vi "Stop Core.vi"(10 "final error code":i32, 11 "DigitiserActor in":refnum<class "DigitiserActor.lvclass">) -> (3 "DigitiserActor out":refnum<class "DigitiserActor.lvclass">)   [LabVIEW 2019, in "DigitiserActor.lvlib" / "DigitiserActor.lvclass"]
doc: "(<B>Filename</B>: Actor Framework.lvlib:Actor.lvclass:Stop Core.vi)\n\nDefines what the actor does before it stops. Use the <B>final error code</B> input to determine whether the actor shut down in response to an error.\n\nBy default, this method passes the Stop message along to all auto-stop nested actors. A descendant class may override this method to define additional behavior, such as shutting down any processes the actor initiated in its override of the Actor Core method."
uses:
  DigitiserActor.lvclass
  <vilib>/ActorFramework/Actor/Actor.lvclass
  <vilib>/ActorFramework/Stop Msg/Stop Msg.lvclass
  C:/Program Files (x86)/National Instruments/LabVIEW 2019/vi.lib/ActorFramework/Actor/Actor.lvclass
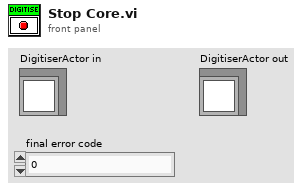
[diagram p1: front panel]
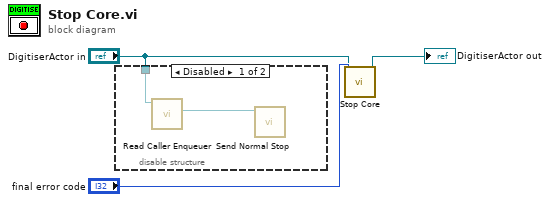
[diagram p0: block diagram]
diagram:
  n1 = disable-structure shown="Disabled" {
    disable-tunnel: "DigitiserActor in" -> [w5 _]
    frame Disabled {
      n2 = call <vilib>:"Read Caller Enqueuer.vi"("Actor"=w5) -> ("Caller Enqueuer"=w4:refnum<class "Message Enqueuer.lvclass">)  [unwired: 10 in]
      n3 = call <vilib>:"Send Normal Stop.vi"("Message Enqueuer"=w4) -> ()  [unwired: 10 in, 1 out]
    }
    frame Enabled {
    }
  }
  n4 = call-parent "Stop Core.vi"("final error code"="final error code", "Actor in"="DigitiserActor in") -> ("Actor out"=→"DigitiserActor out":refnum<class "DigitiserActor.lvclass">)  [unwired: 9 in]
